vi "UpdateiSpkEn.vi"(7 "LabVIEW Web Service Request":refnum<class "Web Request.lvclass">, 11 "iSpkEnByte":u8) -> ()   [LabVIEW 2014]
uses:
  <vilib>/wsapi/Web Request.lvclass
  Controller/Controls/Enqueuer Enum.ctl
  Instr Actor/Messages/Set iSpkEn MSG/Set iSpkEn MSG.lvclass
  Instr Actor/Messages/Set iSpkEn MSG/Set iSpkEn MSG.lvclass/Set iSpkEn MSG.ctl
  Controller/Controller.lvclass
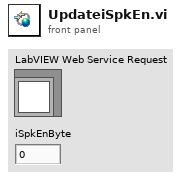
[diagram p1: front panel]
types:
  T1 = typedef "Controller.lvlib/Controller.lvclass/Enqueuer Enum.ctl" = enum8{"PAS", "CRDS", "File", "O3Lamp"}
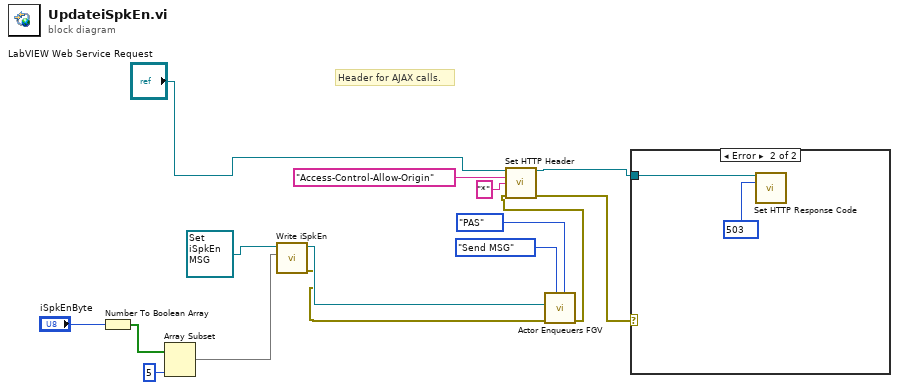
[diagram p0: block diagram]
diagram:
  # "Header for AJAX calls."
  n1 = Number To Boolean Array(number="iSpkEnByte") -> (Boolean array=w12:bool[])
  n2 = Array Subset(array=w12, length=5) -> (w9:bool[])  [unwired: 1 in]
  n3 = call "Write iSpkEn.vi"("iSpkEn"=w9, "Set iSpkEn MSG in"=refnum<class "Set iSpkEn MSG.lvclass"> refnum ("Instrument Lib:Set iSpkEn MSG.lvclass")) -> ("error out"=w7:errorcluster, "Set iSpkEn MSG out"=w8:refnum<class "Set iSpkEn MSG.lvclass">)  [unwired: 8 in]
  n4 = call "Actor Enqueuers FGV.vi"("Enqueuer"=Enqueuer_Enum."PAS", "State"=enum16{"Store", "Send MSG"}."Send MSG", "error in"=w7, "MSG"=w8) -> ("error out"=w2:errorcluster)  [unwired: 7 in]
  n5 = call <vilib>:"Set HTTP Header.vi"("LabVIEW Web Service Request"="LabVIEW Web Service Request", "header"="Access-Control-Allow-Origin", "header value"="*", "error in (no error)"=w2) -> ("LabVIEW Web Service Request out"=w3:refnum<class "Web Request.lvclass">, "error out"=w1:errorcluster)  [unwired: 10 in]
  n6 = case shown="Error" w1 {
    tunnel: w3 -> [_ w16]
    frame No Error {
    }
    frame Error {
      w17 = 503 items=["100"=100, "101"=101, "200"=200, "201"=201, "202"=202, "203"=203, "204"=204, "205"=205, "206"=206, "300"=300, "301"=301, "302"=302, "303"=303, "304"=304, "305"=305, "306"=306, "307"=307, "400"=400, "401"=401, "402"=402, "403"=403, "404"=404, "405"=405, "406"=406, "407"=407, "408"=408, "409"=409, "410"=410, "411"=411, "412"=412, "413"=413, "414"=414, "415"=415, "416"=416, "417"=417, "500"=500, "501"=501, "502"=502, "503"=503, "504"=504, "505"=505] ("response code (200)")
      n7 = call <vilib>:"Set HTTP Response Code.vi"("LabVIEW Web Service Request"=w16, "response code (200)"=w17) -> ()  [unwired: 12 in, 2 out]
    }
  }
